vi "类型1自动误差计算.vi"(8 "允许误差":dbl, 9 "模拟量量程范围":dbl, 10 "设定值_1":dbl, 11 "反馈值_1":dbl) -> (1 "字符串_误差_1":string, 2 "误差_1":dbl, 3 "合格_1?":bool)   [LabVIEW 2010]
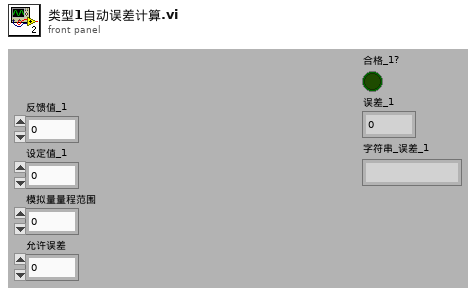
[diagram p1: front panel]
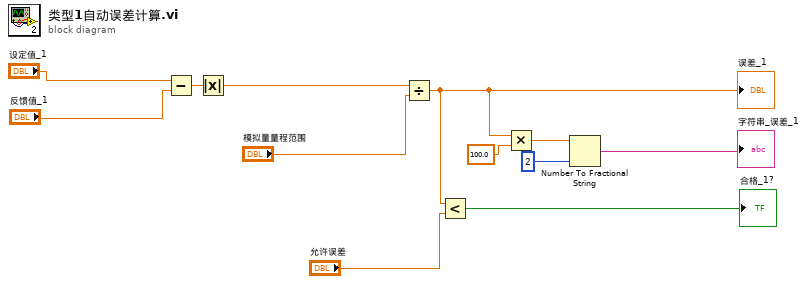
[diagram p0: block diagram]
diagram:
  n1 = Subtract(x="设定值_1", y="反馈值_1") -> (x-y=w12:dbl)
  n2 = Absolute Value(x=w12) -> (abs(x)=w10:dbl)
  n3 = Divide(x=w10, y="模拟量量程范围") -> (x/y=w6:dbl)
  "误差_1" <- w6
  n4 = Less?(x=w6, y="允许误差") -> (x < y?=→"合格_1?":bool)
  n5 = Multiply(x=w6, y=100.0) -> (x*y=w7:dbl)
  n6 = Number To Fractional String(number=w7, precision (6)=i16 2 ("精度(6)")) -> (F-format string=→"字符串_误差_1":string)  [unwired: 2 in]
